vi "Initialize Configuration DVR.vi"(11 "Rename As Application UI Configuration":T1) -> ()   [LabVIEW 2020, in "Performance Monitor UI.lvlib" / "Configuration.lvlib"]
doc: "Initialize the Configuration DVR global. This is the only place where the global is written...on DVR initialization.\n_____\nBased on DCFG Project Template 1.0.0.21.\n____\nPeloton Config 1.0.0.2\nCopyright (c) 2022, Peloton"
uses:
  Configuration.lvlib
  Configuration--cluster.ctl
  Configuration DVR Global.vi
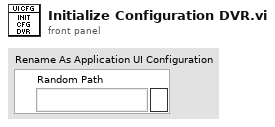
[diagram p1: front panel]
types:
  T1 = typedef "Performance Monitor UI.lvlib/Configuration.lvlib/Configuration--cluster.ctl" = cluster{"Random Path":path}
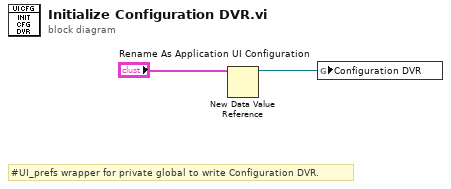
[diagram p0: block diagram]
diagram:
  # "#UI_prefs wrapper for private global to write Configuration DVR."
  n1 = New Data Value Reference(data value="Rename As Application UI Configuration") -> (data value reference=w1:refnum<data-value>)  [unwired: 1 in, 1 out]
  n2 = global write "Configuration DVR Global.vi" "Configuration DVR"(w1) -> ()
